vi "Ignore-error-multiple.vi"(8 "error in (no error)":errorcluster, 10 "Errors to ignore":i32[](array[numeric])) -> (0 "error out":errorcluster)   [LabVIEW 2013, in "Error-handling.lvlib" / "Errors.lvclass"]
uses:
  Errors.lvclass
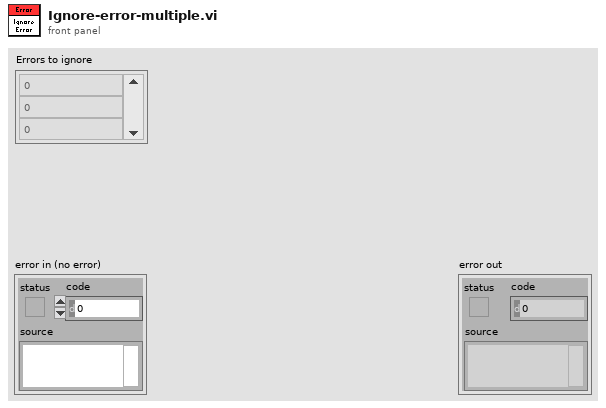
[diagram p1: front panel]
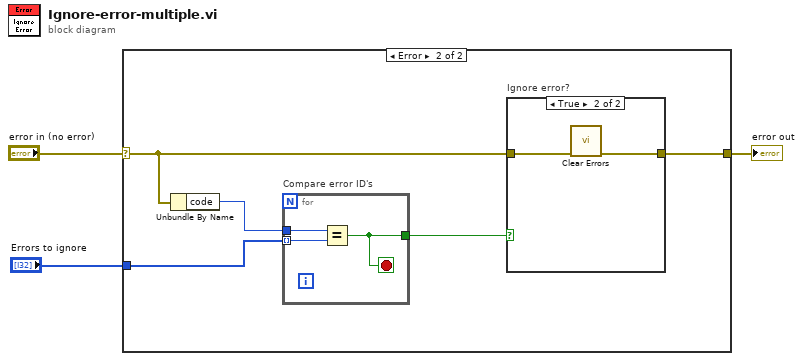
[diagram p0: block diagram]
diagram:
  n1 = case shown="Error" "error in (no error)" {
    selector: "error in (no error)" -> [w4 w6]
    tunnel: [w4 w5] -> w2
    tunnel: "Errors to ignore" -> [_ w8]
    frame No Error {
    }
    frame Error {
      n2 = Unbundle By Name(w6) -> ("code"=w9:i32)
      n3 = for "Compare error ID's" {
        tunnel: w9 -> [w12]
        tunnel: w8 -> [w11] mode=indexing
        tunnel: [w10] -> w7
        stop <- w10 stop-if-true
        n4 = Equal?(x=w12, y=w11) -> (x = y?=w10:bool)
      }
      n5 = case "Ignore error?" shown="True" w7 {
        tunnel: w6 -> [w13 w15]
        tunnel: [w13 w14] -> w5
        frame False {
        }
        frame True {
          n6 = call <vilib>:"Clear Errors.vi"("error in (no error)"=w15) -> ("error out"=w14:errorcluster)  [unwired: 6 in]
        }
      }
    }
  }
  "error out" <- w2
